vi "ApostrophString.vi"(11 "String in":string) -> (3 "String out":string)   [LabVIEW 2013, in "main.lvlib"]
uses:
  main.lvlib
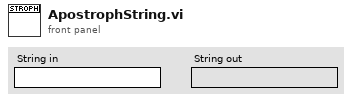
[diagram p1: front panel]
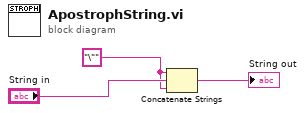
[diagram p0: block diagram]
diagram:
  w1 = "\""
  n1 = Concatenate Strings(w1, "String in", w1) -> (→"String out":string)
